vi "Actor Core.vi"(8 "error in":errorcluster, 11 "Measurement in":refnum<class "Measurement.lvclass">) -> (0 "error out":errorcluster, 3 "Actor out":refnum<class "Actor.lvclass">)   [LabVIEW 2020, in "Measurement.lvlib" / "Measurement.lvclass"]
doc: "(<B>Filename</B>: Actor Framework.lvlib:Actor.lvclass:Actor Core.vi)\n\nReceives messages to the actor, reacts to them, and initiates any error handling that may shut the actor down.\n\nDescendant classes may override this VI to append parallel tasks for the actor to complete while it handles messages. Overrides use the Call Parent Class Method node."
uses:
  Measurement.lvclass
  C:/Program Files/National Instruments/LabVIEW 2020/vi.lib/ActorFramework/Actor/Actor.lvclass
  <vilib>/ActorFramework/Actor/Actor.lvclass
  <vilib>/ActorFramework/Actor/Actor.lvclass/Actor.ctl
  Measurement.lvclass/Measurement.ctl
  GUI_Graph Messages/Graph Data Msg/Graph Data Msg.lvclass/Graph Data Msg.ctl
  <vilib>/ActorFramework/Message Enqueuer/Message Enqueuer.lvclass/Message Enqueuer.ctl
  <vilib>/ActorFramework/Message Enqueuer/Enqueue.vi
  GUI_Graph Messages/Graph Data Msg/Graph Data Msg.lvclass
  C:/Program Files/National Instruments/LabVIEW 2020/vi.lib/ActorFramework/Message/Message.lvclass
  <vilib>/ActorFramework/Message Priority Queue/Priority Enqueue.vi
  <vilib>/measure/NI_MABase.lvlib
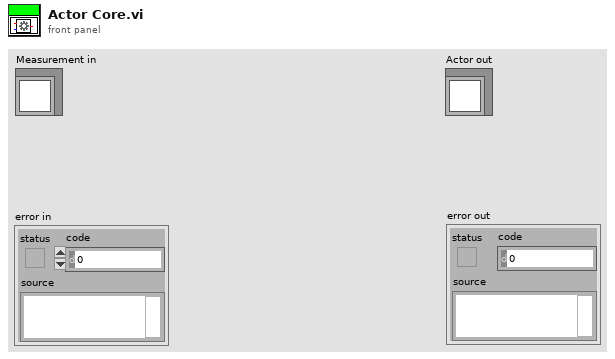
[diagram p1: front panel]
types:
  T1 = cluster{"Start/stop HL":refnum<user-event>, "Exit":refnum<user-event>, "Amplitud":refnum<user-event>, "Frecuencia":refnum<user-event>, "signal":refnum<user-event>}
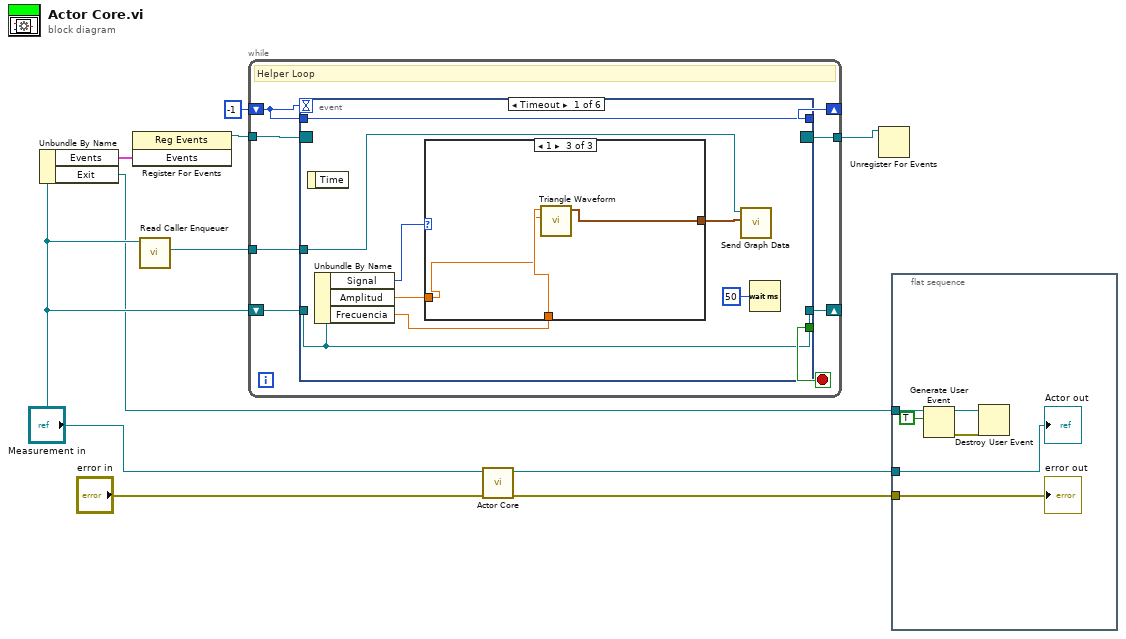
[diagram p0: block diagram]
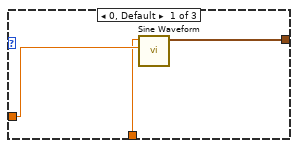
[diagram p2: hidden frame]
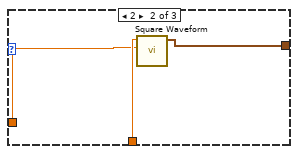
[diagram p3: hidden frame]
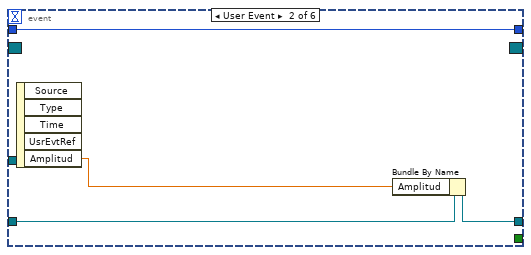
[diagram p4: hidden frame]
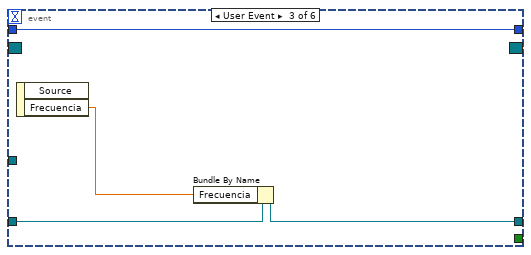
[diagram p5: hidden frame]
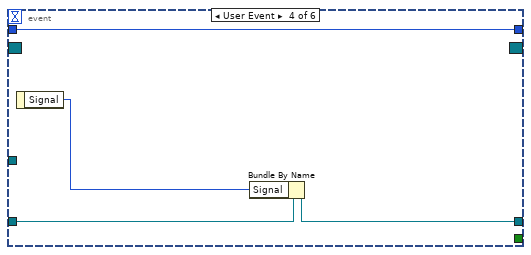
[diagram p6: hidden frame]
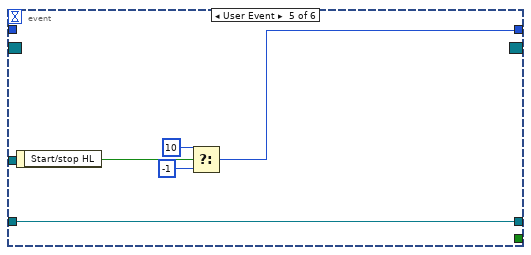
[diagram p7: hidden frame]
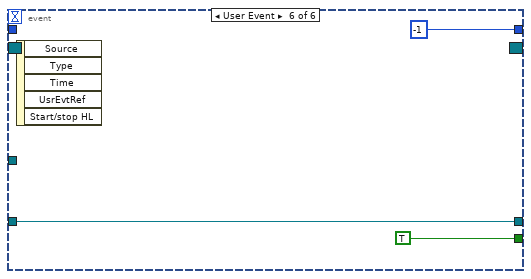
[diagram p8: hidden frame]
diagram:
  n1 = Unbundle By Name("Measurement in") -> ("Events"=w7:T1, "Exit"=w2:refnum<user-event>)
  n2 = register-events(w7) -> (reference out=w6:refnum<event-registration>)  [unwired: 2 in, 1 out]
  n3 = call <vilib>:"Read Caller Enqueuer.vi"("Actor"="Measurement in") -> ("Caller Enqueuer"=w5:refnum<class "Message Enqueuer.lvclass">)  [unwired: 10 in]
  n4 = while {
    tunnel: w6 -> [w15]
    tunnel: w5 -> [w18]
    shift-right: [w16] -> _
    shift-left: "Measurement in" -> [w17]
    shift-right: [w14] -> _
    shift-left: -1 -> [w13]
    tunnel: [w11] -> w1
    stop <- w12 stop-if-true
    # "Helper Loop"
    n5 = event shown="[0] Timeout" {
      selector: w15 -> [_ _ _ _ _ _]
      dyn-events: [_ _ _ _ _ _] -> w11
      timeout: w13 -> [_ _ _ _ _ _]
      tunnel: w18 -> [w21 _ _ _ _ _]
      tunnel: w17 -> [w25 w39 w43 w47 w48 w53]
      tunnel: [w25 w38 w42 w46 w48 w53] -> w16
      tunnel: w13 -> [w26 w36 w40 w44 _ _]
      tunnel: [w26 w36 w40 w44 w49 -1 ("f")] -> w14
      tunnel: [_ _ _ _ _ TRUE] -> w12
      event Timeout {
        n6 = event-data() -> ()  [unwired: 1 in, 1 out]
        n7 = Unbundle By Name(w25) -> ("Signal"=w24:u16, "Amplitud"=w23:dbl, "Frecuencia"=w22:dbl)
        n8 = case shown="1" w24 {
          tunnel: w23 -> [w29 w31 w34]
          tunnel: w22 -> [w28 w32 w35]
          tunnel: [w27 w30 w33] -> w20
          frame 0, Default {
            n9 = call <vilib>:"Sine Waveform.vi"("amplitude"=w29, "frequency"=w28) -> ("signal out"=w27:waveform(dbl))  [unwired: 8 in, 1 out]
          }
          frame 2 {
            n10 = call <vilib>:"Square Waveform.vi"("amplitude"=w31, "frequency"=w32) -> ("signal out"=w30:waveform(dbl))  [unwired: 8 in, 1 out]
          }
          frame 1 {
            n11 = call <vilib>:"Triangle Waveform.vi"("amplitude"=w34, "frequency"=w35) -> ("signal out"=w33:waveform(dbl))  [unwired: 8 in, 1 out]
          }
        }
        n12 = call "Send Graph Data.vi"("signal out"=w20, "Message Enqueuer"=w21) -> ()  [unwired: 8 in, 2 out]
        n13 = Wait (ms)(milliseconds to wait=u32 50) -> ()  [unwired: 1 out]
      }
      event User Event {
        n14 = event-data() -> ("Amplitud"=w37:dbl)  [unwired: 1 in, 4 out]
        n15 = Bundle By Name(cluster=w39, "Amplitud"=w37) -> (w38:refnum<class "Measurement.lvclass">)
      }
      event User Event {
        n16 = event-data() -> ("Frecuencia"=w41:dbl)  [unwired: 1 in, 1 out]
        n17 = Bundle By Name(cluster=w43, "Frecuencia"=w41) -> (w42:refnum<class "Measurement.lvclass">)
      }
      event User Event {
        n18 = event-data() -> ("Signal"=w45:u16)  [unwired: 1 in]
        n19 = Bundle By Name(cluster=w47, "Signal"=w45) -> (w46:refnum<class "Measurement.lvclass">)
      }
      event User Event {
        n20 = event-data() -> ("Start/stop HL"=w52:bool)  [unwired: 1 in]
        n21 = Select(t=10, s=w52, f=-1) -> (s? t:f=w49:i32)
      }
      event User Event {
        n22 = event-data() -> ()  [unwired: 1 in, 5 out]
      }
    }
  }
  n23 = call-parent "Actor Core.vi"("error in"="error in", "Actor in"="Measurement in") -> ("error out"=w10:errorcluster, "Actor out"=w9:refnum<class "Actor.lvclass">)  [unwired: 8 in]
  n24 = Unregister For Events(event registration refnum=w1) -> ()  [unwired: 1 in, 1 out]
  n25 = flat-sequence {
    tunnel: w10 -> [w61]
    tunnel: w9 -> [w60]
    tunnel: w2 -> [w59]
    frame #0 {
      n26 = Generate User Event(user event=w59, event data cluster=TRUE ("event data")) -> (user event out=w56:refnum<user-event>, error out=w57:errorcluster)  [unwired: 2 in]
      n27 = Destroy User Event(user event=w56, error in=w57) -> ()  [unwired: 1 out]
      "error out" <- w61
      "Actor out" <- w60
    }
  }
